vi "PID Integral Control start.vi"(0 "Temp In (deg C)":dbl format="%.2f", 2 "in control band":bool, 7 "Control Parameters":T1={"Setpoint"=50.0, "Control Bandwidth"=4.0, "Integral Time"=30.0, "Int\nON"=TRUE, "Derivative Tme"=0.5, "Der\nON"=TRUE, "Settle Bandwidth"=1.0, "Settle Time"=200.0} {"Settle Time" step=1.0; "Settle Bandwidth" step=0.01; "Derivative Tme" step=0.01; "Integral Time" step=1.0; "Control Bandwidth" step=0.1; "Setpoint" step=0.1}, 9 "reset":bool, 11 "delta t":dbl format="%.2f") -> (8 "Integral Power":dbl format="%.2f")   [LabVIEW 2019]
doc: "Subvi \n\nThis does the integral part of the PID controller \nalso deals with intergral windup\n\nJuan Gamez\nP3600\nCSUSB"
uses:
  typedefs/PID control parameters.ctl
panel:
  # "PID\nIntegral\nPower\nControl"
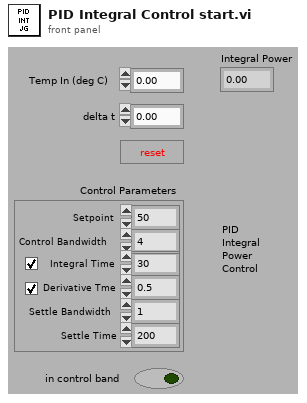
[diagram p1: front panel]
types:
  T1 = typedef "PID control parameters.ctl" = cluster{"Setpoint":dbl, "Control Bandwidth":dbl, "Integral Time":dbl, "Int\nON":bool, "Derivative Tme":dbl, "Der\nON":bool, "Settle Bandwidth":dbl, "Settle Time":dbl}
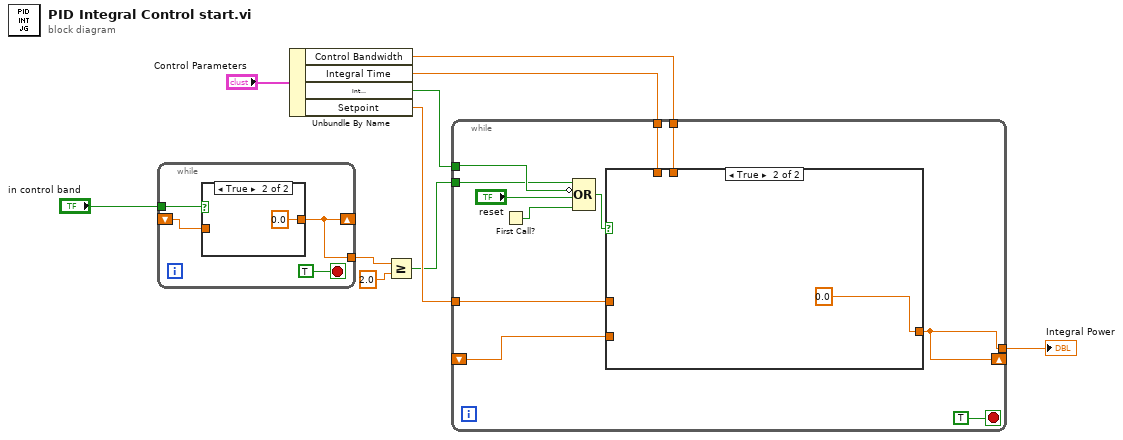
[diagram p0: block diagram]
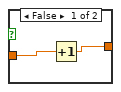
[diagram p2: hidden frame]
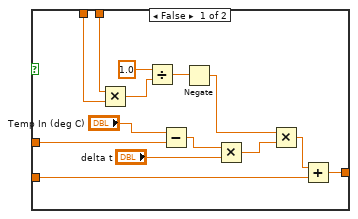
[diagram p3: hidden frame]
diagram:
  n1 = while {
    shift-right: [w12] -> _
    shift-left: _ -> [w14]
    tunnel: "in control band" -> [w13]
    tunnel: [w12] -> w5
    stop <- TRUE stop-if-true
    n2 = case shown="True" w13 {
      tunnel: w14 -> [w16 _]
      tunnel: [w15 0.0] -> w12
      frame False {
        n3 = Increment(x=w16) -> (x+1=w15:dbl)
      }
      frame True {
      }
    }
  }
  n4 = Unbundle By Name("Control Parameters") -> ("Control Bandwidth"=w2:dbl, "Integral Time"=w1:dbl, "Int\nON"=w9:bool, "Setpoint"=w8:dbl)
  n5 = Greater Or Equal?(x=w5, y=2.0) -> (x >= y?=w4:bool)
  n6 = while {
    tunnel: w9 -> [w24]
    shift-right: [w20] -> _
    shift-left: _ -> [w21]
    tunnel: w8 -> [w25]
    tunnel: w4 -> [w22]
    tunnel: [w20] -> w3
    tunnel: w2 -> [w19]
    tunnel: w1 -> [w18]
    stop <- TRUE stop-if-true
    n7 = First Call?() -> (First Call?: T/F=w27:bool)
    n8 = Compound Arithmetic op=OR(w22, invert w24, "reset", w27) -> (w26:bool)
    n9 = case shown="True" w26 {
      tunnel: w25 -> [w38 _]
      tunnel: w21 -> [w33 _]
      tunnel: [w32 0.0] -> w20
      tunnel: w19 -> [w30 _]
      tunnel: w18 -> [w29 _]
      frame False {
        n10 = Multiply(x=w30, y=w29) -> (x*y=w42:dbl)
        n11 = Divide(x=1.0, y=w42) -> (x/y=w40:dbl)
        n12 = Subtract(x="Temp In (deg C)", y=w38) -> (x-y=w36:dbl)
        n13 = Negate(x=w40) -> (-x=w35:dbl)
        n14 = Multiply(x=w36, y="delta t") -> (x*y=w34:dbl)
        n15 = Multiply(x=w35, y=w34) -> (x*y=w31:dbl)
        n16 = Add(x=w31, y=w33) -> (x+y=w32:dbl)
      }
      frame True {
      }
    }
  }
  "Integral Power" <- w3
